vi "Handle Player.vi"(6 "Apply?":bool, 7 "p":i32, 9 "Additional Wait":i32, 10 "Data":T1) -> (1 "Output":T5, 2 "Data out":T1)   [LabVIEW 2015, in "TeamEffort.lvclass"]
uses:
  TeamEffort.lvclass
  Grid Cluster.ctl
  Player Cluster.ctl
  Square/Square.lvclass
  Team Move Input.ctl
  Type Defs/Action Enum.ctl
  Team Move Output.ctl
  Type Defs/Direction Enum.ctl
  Type Defs/SB Type Defs.lvlib
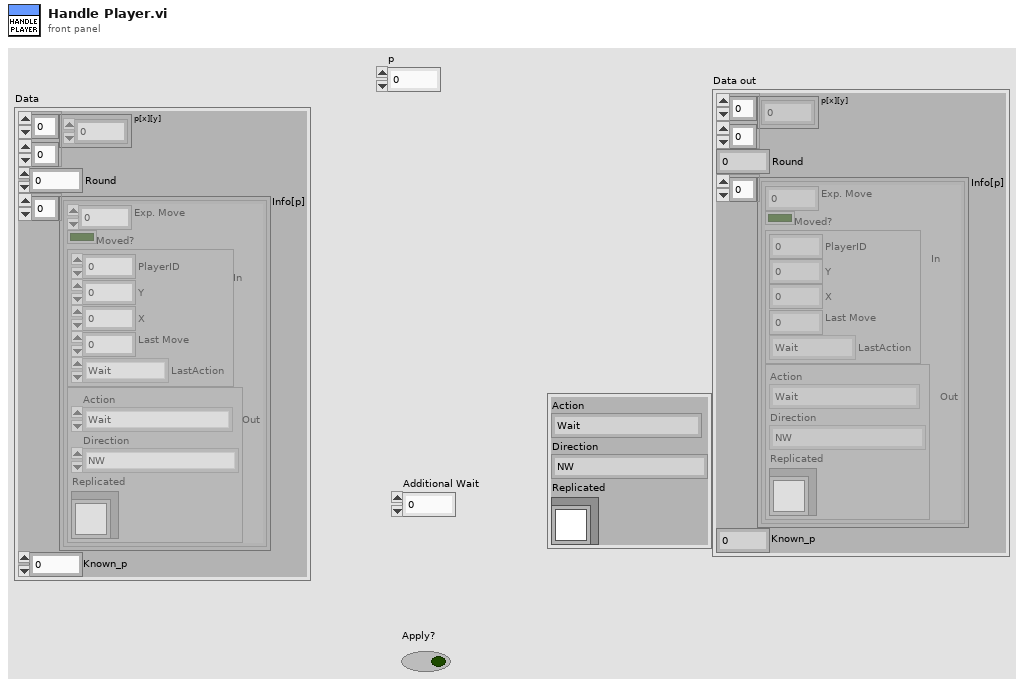
[diagram p1: front panel]
types:
  T1 = typedef "TeamEffort.lvclass/Grid Cluster.ctl" = cluster{"p[x][y]":i32[][], "Round":i32, "Info[p]":T2[], "Known_p":i32}
  T2 = typedef "TeamEffort.lvclass/Player Cluster.ctl" = cluster{"Exp. Move":i32, "Moved?":bool, "In":T3, "Out":T5}
  T3 = typedef "TeamEffort.lvclass/Team Move Input.ctl" = cluster{"PlayerID":i32, "Y":i32, "X":i32, "Last Move":i32, "LastAction":T4}
  T4 = typedef "SB Type Defs.lvlib/Action Enum.ctl" = enum16{"Wait", "Move", "Attack", "Replicate"}
  T5 = typedef "TeamEffort.lvclass/Team Move Output.ctl" = cluster{"Action":T4, "Direction":T6, "Replicated":refnum<class "Square.lvclass">}
  T6 = typedef "SB Type Defs.lvlib/Direction Enum.ctl" = enum16{"NW", "N", "NE", "E", "SE", "S", "SW", "W"}
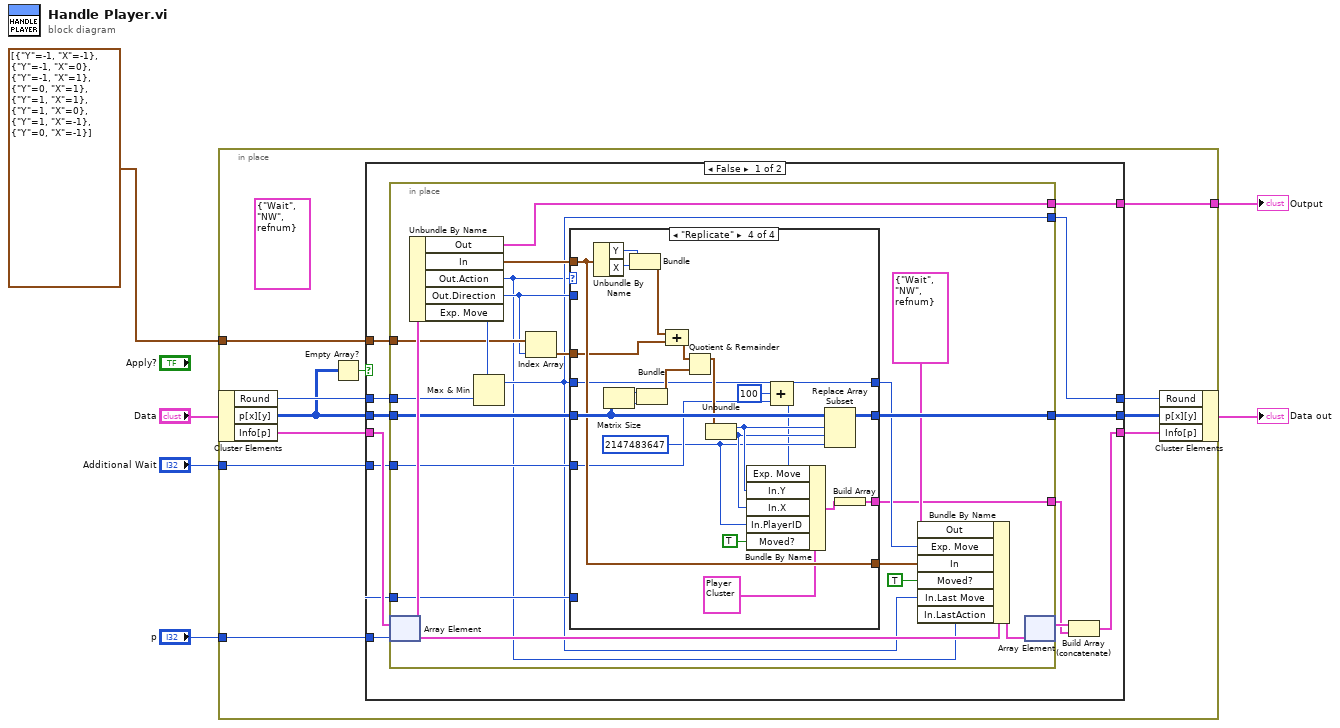
[diagram p0: block diagram]
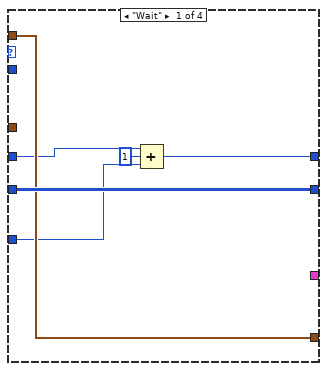
[diagram p2: hidden frame]
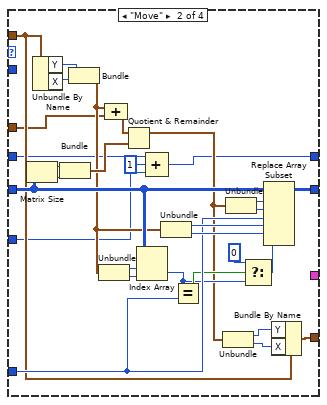
[diagram p3: hidden frame]
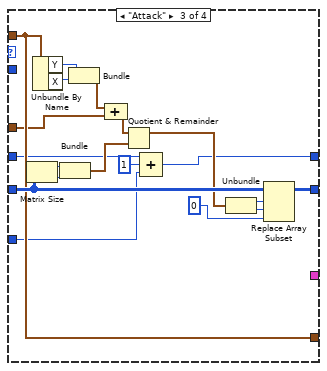
[diagram p4: hidden frame]
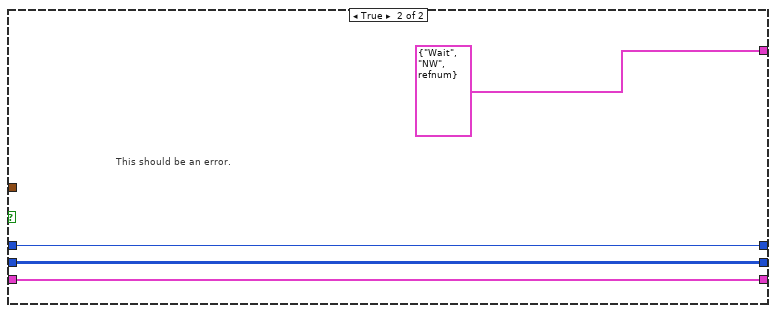
[diagram p5: hidden frame]
diagram:
  n1 = in-place {
    in-place-border: "p" -> [w12]
    in-place-border: [w15] -> w4
    in-place-border: cluster{"Y":i32, "X":i32}[] [{"Y"=-1, "X"=-1}, {"Y"=-1, "X"=0}, {"Y"=-1, "X"=1}, {"Y"=0, "X"=1}, {"Y"=1, "X"=1}, {"Y"=1, "X"=0}, {"Y"=1, "X"=-1}, {"Y"=0, "X"=-1}] -> [w11]
    in-place-border: "Additional Wait" -> [w10]
    (unwired) T5 {"Action"=enum."Wait", "Direction"=enum."NW", "Replicated"=refnum} ("Output")
    n2 = in-place-cluster #1("Data") -> ("Round"=w16:i32, "p[x][y]"=w7:i32[][], "Info[p]"=w17:T2[])
    n3 = Empty Array?(array=w7) -> (empty?=w8:bool)
    n4 = case shown="False" w8 {
      tunnel: w17 -> [w29 w129]
      tunnel: w16 -> [w28 w130]
      tunnel: [w27 T5 {"Action"=enum."Wait", "Direction"=enum."NW", "Replicated"=refnum} ("Out")] -> w15
      tunnel: [w26 w130] -> w14
      tunnel: [w24 w131] -> w13
      tunnel: w12 -> [w23 _]
      tunnel: w11 -> [w22 _]
      tunnel: w10 -> [w21 _]
      tunnel: [w20 w129] -> w9
      tunnel: w7 -> [w18 w131]
      frame False {
        n5 = in-place {
          in-place-border: w28 -> [w45]
          in-place-border: [w31] -> w26
          in-place-border: w18 -> [w44]
          in-place-border: [w43] -> w24
          in-place-border: [w40] -> w27
          in-place-border: w23 -> [w38]
          in-place-border: w22 -> [w37]
          in-place-border: w21 -> [w34]
          in-place-border: [w32] -> w19
          n6 = in-place-array #2(w29, w23) -> (w47:T2)
          n7 = Unbundle By Name(w47) -> ("Out"=w40:T5, "In"=w39:T3, "Out.Action"=w30:T4, "Out.Direction"=w36:T6, "Exp. Move"=w46:i32)
          n8 = Max & Min(x=w46, y=w45) -> (max(x,y)=w31:i32)  [unwired: 1 out]
          n9 = Index Array(array=w37, index=w36) -> (element=w35:cluster{"Y":i32, "X":i32})
          n10 = case shown="\"Replicate\"" w30 {
            tunnel: w44 -> [w55 w85 w104 w127]
            tunnel: [w55 w78 w97 w120] -> w43
            tunnel: w31 -> [w53 w59 w89 w115]
            tunnel: [w50 w57 w88 w105] -> w41
            tunnel: [w54 w63 w91 w118] -> w42
            tunnel: w39 -> [w54 w64 w91 w118]
            tunnel: w36 -> [_ _ _ _]
            tunnel: w38 -> [_ w68 _ _]
            tunnel: w35 -> [_ w60 w90 w116]
            tunnel: w34 -> [w52 w58 w87 w113]
            tunnel: [_ _ _ w106] -> w32
            frame "Wait" {
              n11 = Compound Arithmetic op=ADD(w53, 1 ("value"), w52) -> (w50:i32)
            }
            frame "Move" {
              n12 = Matrix Size(0:w85) -> (1:w84:i32, 2:w83:i32)
              n13 = Unbundle By Name(w64) -> ("Y"=w81:i32, "X"=w82:i32)
              n14 = Bundle("number of columns"=w84, "matrix"=w83) -> (w79:cluster{"number of columns":i32, "matrix":i32})  [unwired: 1 in]
              n15 = Bundle("Y"=w81, "X"=w82) -> (w73:cluster{"Y":i32, "X":i32})  [unwired: 1 in]
              n16 = Unbundle(w73) -> ("Y"=w75:i32, "X"=w74:i32)
              n17 = Compound Arithmetic op=ADD(w73, w60) -> (w80:cluster{"Y":i32, "X":i32})
              n18 = Quotient & Remainder(x=w80, y=w79) -> (x-y*floor(x/y)=w65:cluster{i32, i32})  [unwired: 1 out]
              n19 = Index Array(array=w85, index (row)=w75, index (col)=w74) -> (element=w66:i32)
              n20 = Compound Arithmetic op=ADD(w59, 1 ("value"), w58) -> (w57:i32)
              n21 = Unbundle(w73) -> ("Y"=w72:i32, "X"=w71:i32)
              n22 = Equal?(x=w66, y=w68) -> (x = y?=w67:bool)
              n23 = Unbundle(w65) -> (w62:i32, w61:i32)
              n24 = Unbundle(w65) -> (w77:i32, w76:i32)
              n25 = Select(t=0, s=w67, f=w66) -> (s? t:f=w70:i32)
              n26 = Replace Array Subset(array=w85, new element #1=w68, index (row) #1=w77, index (col) #1=w76, new element #2=w70, index (row) #2=w72, index (col) #2=w71) -> (w78:i32[][])
              n27 = Bundle By Name(cluster=w64, "Y"=w62, "X"=w61) -> (w63:T3)
            }
            frame "Attack" {
              n28 = Matrix Size(0:w104) -> (1:w103:i32, 2:w102:i32)
              n29 = Unbundle By Name(w91) -> ("Y"=w100:i32, "X"=w101:i32)
              n30 = Bundle("number of columns"=w103, "matrix"=w102) -> (w98:cluster{"number of columns":i32, "matrix":i32})  [unwired: 1 in]
              n31 = Bundle("Y"=w100, "X"=w101) -> (w94:cluster{"Y":i32, "X":i32})  [unwired: 1 in]
              n32 = Compound Arithmetic op=ADD(w94, w90) -> (w99:cluster{"Y":i32, "X":i32})
              n33 = Quotient & Remainder(x=w99, y=w98) -> (x-y*floor(x/y)=w93:cluster{i32, i32})  [unwired: 1 out]
              n34 = Compound Arithmetic op=ADD(w89, 1 ("value"), w87) -> (w88:i32)
              n35 = Unbundle(w93) -> (w96:i32, w95:i32)
              n36 = Replace Array Subset(array=w104, new element=0 ("new element/subarray"), index (row)=w96, index (col)=w95) -> (w97:i32[][])
            }
            frame "Replicate" {
              w110 = 2147483647 ("new element/subarray")
              n37 = Unbundle By Name(w118) -> ("Y"=w123:i32, "X"=w124:i32)
              n38 = Matrix Size(0:w127) -> (1:w126:i32, 2:w125:i32)
              n39 = Bundle("Y"=w123, "X"=w124) -> (w119:cluster{"Y":i32, "X":i32})  [unwired: 1 in]
              n40 = Bundle("number of columns"=w126, "matrix"=w125) -> (w121:cluster{"number of columns":i32, "matrix":i32})  [unwired: 1 in]
              n41 = Compound Arithmetic op=ADD(w119, w116) -> (w122:cluster{"Y":i32, "X":i32})
              n42 = Quotient & Remainder(x=w122, y=w121) -> (x-y*floor(x/y)=w117:cluster{i32, i32})  [unwired: 1 out]
              n43 = Unbundle(w117) -> (w112:i32, w111:i32)
              n44 = Compound Arithmetic op=ADD(w115, 100 ("value"), w113) -> (w105:i32)
              n45 = Bundle By Name(cluster=T2 {"Exp. Move"=0, "Moved?"=FALSE, "In"={"PlayerID"=0, "Y"=0, "X"=0, "Last Move"=0, "LastAction"=enum."Wait"}, "Out"={"Action"=enum."Wait", "Direction"=enum."NW", "Replicated"=refnum}} ("element"), "Exp. Move"=w105, "In.Y"=w112, "In.X"=w111, "In.PlayerID"=w110, "Moved?"=TRUE) -> (w107:T2)
              n46 = Replace Array Subset(array=w127, new element=w110, index (row)=w112, index (col)=w111) -> (w120:i32[][])
              n47 = Build Array(w107) -> (w106:T2[])
            }
          }
          n48 = Bundle By Name(cluster=w47, "Out"=T5 {"Action"=enum."Wait", "Direction"=enum."NW", "Replicated"=refnum}, "Exp. Move"=w41, "In"=w42, "Moved?"=TRUE, "In.Last Move"=w31, "In.LastAction"=w30) -> (w48:T2)
          n49 = in-place-array #2(w48) -> (w25:T2[])  [unwired: 1 out]
        }
        n50 = Build Array (concatenate)(w25, w19) -> (w20:T2[])
      }
      frame True {
        # "This should be an error."
      }
    }
    n51 = in-place-cluster #1("Round"=w14, "p[x][y]"=w13, "Info[p]"=w9) -> (→"Data out":T1)
  }
  "Output" <- w4
